vi "mTTOunit.vi"(5 "Numeric":dbl, 7 "Unit":T1, 11 "error in (no error)":errorcluster) -> (6 "Numeric 2":dbl, 8 "Display":string, 15 "error out":errorcluster)   [LabVIEW 2014, in "FH 55.lvlib"]
uses:
  FH 55.lvlib
  TypeDef/Unit.ctl
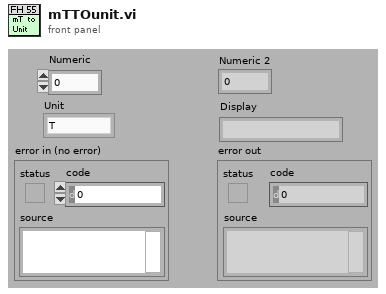
[diagram p1: front panel]
types:
  T1 = typedef "FH 55.lvlib/Unit.ctl" = enum16{"T", "G", "A/m"}
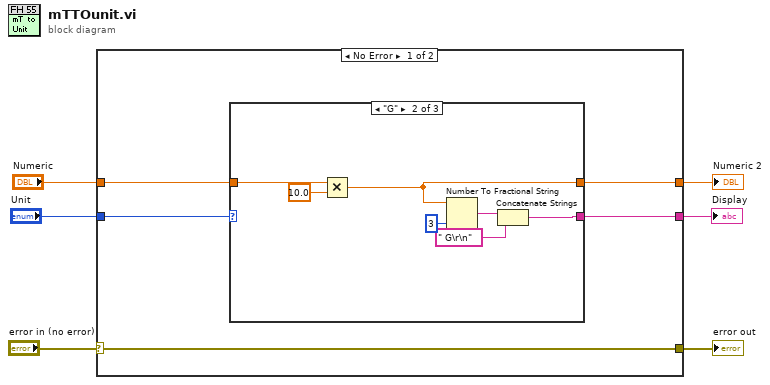
[diagram p0: block diagram]
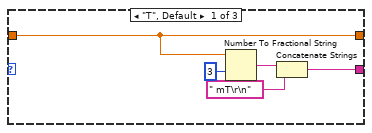
[diagram p2: hidden frame]
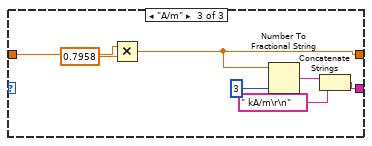
[diagram p3: hidden frame]
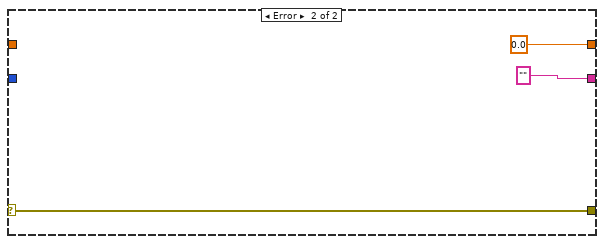
[diagram p4: hidden frame]
diagram:
  n1 = case shown="No Error" "error in (no error)" {
    selector: "error in (no error)" -> [w7 w33]
    tunnel: [w7 w33] -> w5
    tunnel: [w9 0.0] -> w4
    tunnel: "Numeric" -> [w10 _]
    tunnel: "Unit" -> [w11 _]
    tunnel: [w8 ""] -> w1
    frame No Error {
      n2 = case shown="\"G\"" w11 {
        tunnel: w10 -> [w13 w23 w30]
        tunnel: [w13 w18 w25] -> w9
        tunnel: [w14 w19 w26] -> w8
        frame "T", Default {
          n3 = Number To Fractional String(number=w13, precision (6)=i16 3) -> (F-format string=w16:string)  [unwired: 2 in]
          n4 = Concatenate Strings(w16, " mT\r\n" ("string")) -> (w14:string)
        }
        frame "G" {
          n5 = Multiply(x=w23, y=10.0) -> (x*y=w18:dbl)
          n6 = Number To Fractional String(number=w18, precision (6)=i16 3) -> (F-format string=w21:string)  [unwired: 2 in]
          n7 = Concatenate Strings(w21, " G\r\n" ("string")) -> (w19:string)
        }
        frame "A/m" {
          n8 = Multiply(x=w30, y=0.7958) -> (x*y=w25:dbl)
          n9 = Number To Fractional String(number=w25, precision (6)=i16 3) -> (F-format string=w28:string)  [unwired: 2 in]
          n10 = Concatenate Strings(w28, " kA/m\r\n" ("string")) -> (w26:string)
        }
      }
    }
    frame Error {
    }
  }
  "error out" <- w5
  "Numeric 2" <- w4
  "Display" <- w1
